vi "Registration FG.vi"(7 "Registration Actions":T1=enum."Destroy", 8 "error in":errorcluster) -> (0 "error out":errorcluster, 3 "notifier out":refnum<notifier>)   [LabVIEW 2015, in "Generic Module Library.lvlib" / "Template G_Module.lvlib"]
uses:
  Template G_Module.lvlib
  Registration Actions.ctl
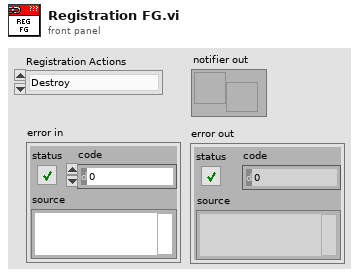
[diagram p1: front panel]
types:
  T1 = typedef "Generic Module Library.lvlib/Template G_Module.lvlib/Registration Actions.ctl" = enum16{"Create", "Get", "Destroy"}
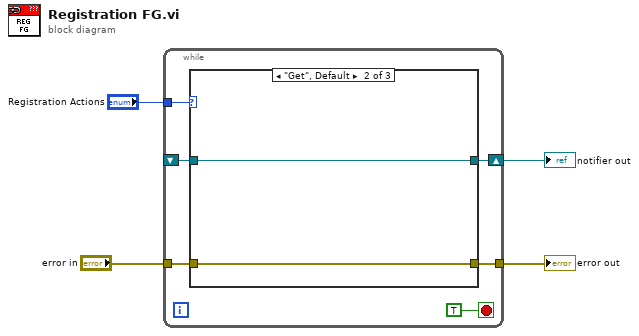
[diagram p0: block diagram]
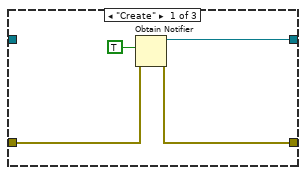
[diagram p2: hidden frame]
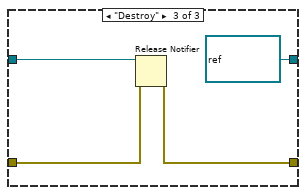
[diagram p3: hidden frame]
diagram:
  n1 = while {
    tunnel: "Registration Actions" -> [w9]
    shift-right: [w8] -> w1
    shift-left: _ -> [w5]
    tunnel: "error in" -> [w7]
    tunnel: [w6] -> w2
    stop <- TRUE stop-if-true
    n2 = case shown="\"Get\", Default" w9 {
      tunnel: [w14 w16 refnum<notifier> refnum ("notifier out")] -> w8
      tunnel: w7 -> [w12 w15 w18]
      tunnel: [w11 w15 w17] -> w6
      tunnel: w5 -> [_ w16 w20]
      frame "Create" {
        n3 = Obtain Notifier(notification data type=TRUE, error in (no error)=w12) -> (notifier out=w14:refnum<notifier>, error out=w11:errorcluster)  [unwired: 2 in, 1 out]
      }
      frame "Get", Default {
      }
      frame "Destroy" {
        n4 = Release Notifier(notifier=w20, error in (no error)=w18) -> (error out=w17:errorcluster)  [unwired: 1 in, 2 out]
      }
    }
  }
  "error out" <- w2
  "notifier out" <- w1
